vi "Assign 3 Washing machine control using basic AND & NOT gates (2).vi"() -> ()   [LabVIEW 2021]
panel:
  out "MOTOR":bool
  out "HEATER":bool
  out "WATER VALVE":bool
  in  "WATER TEMP SENSOR":bool
  in  "WATER LEVEL SENSOR":bool
  in  "DOOR SENSOR":bool
  # "Sagar C V"
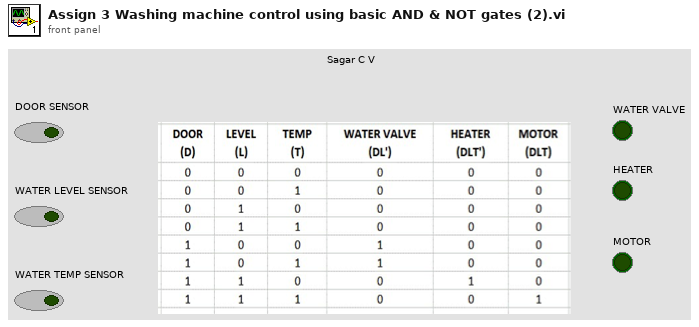
[diagram p1: front panel]
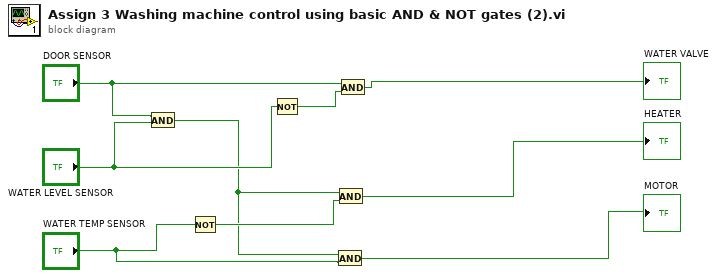
[diagram p0: block diagram]
diagram:
  n1 = And(x="DOOR SENSOR", y="WATER LEVEL SENSOR") -> (x .and. y?=w3:bool)
  n2 = Not(x="WATER TEMP SENSOR") -> (.not. x?=w4:bool)
  n3 = Not(x="WATER LEVEL SENSOR") -> (.not. x?=w9:bool)
  n4 = And(x=w3, y="WATER TEMP SENSOR") -> (x .and. y?=→"MOTOR":bool)
  n5 = And(x=w3, y=w4) -> (x .and. y?=→"HEATER":bool)
  n6 = And(x="DOOR SENSOR", y=w9) -> (x .and. y?=→"WATER VALVE":bool)
